vi "WriteBin.vi"() -> ()   [LabVIEW 2014]
panel:
  out "number (0 to 1)":dbl
  in  "Path":path
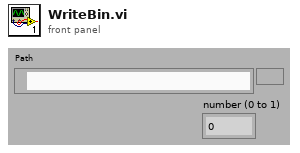
[diagram p1: front panel]
types:
  T1 = enum16{"open", "replace", "create", "open or create", "replace or create", "replace or create with confirmation"}
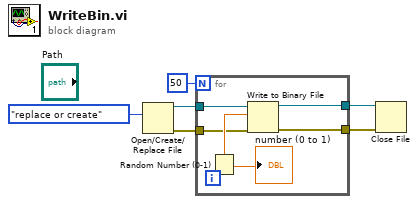
[diagram p0: block diagram]
diagram:
  n1 = Open/Create/Replace File(operation (0:open)=T1."replace or create") -> (refnum out=w5:refnum<file>, error out=w4:errorcluster)  [unwired: 5 in, 1 out]
  n2 = for {
    N: 50 -> [_]
    tunnel: w5 -> [w11]
    tunnel: w4 -> [w8]
    tunnel: [w10] -> w3
    tunnel: [w7] -> w1
    n3 = Random Number (0-1)() -> (number: 0 to 1=w9:dbl)
    "number (0 to 1)" <- w9
    n4 = Write to Binary File(file (use dialog)=w11, data=w9, error in=w8) -> (refnum out=w10:refnum<file>, error out=w7:errorcluster)  [unwired: 3 in, 1 out]
  }
  n5 = Close File(refnum=w3, error in=w1) -> ()  [unwired: 2 out]
